vi "CreatActivationCode.vi"() -> ()   [LabVIEW 2018]
panel:
  in  "生成":bool
  in  "激活码":string
  in  "MAC":string
  in  "使用期限":timestamp=timestamp(3629145600 s since 1904-01-01) format="%<%Y%m>T"
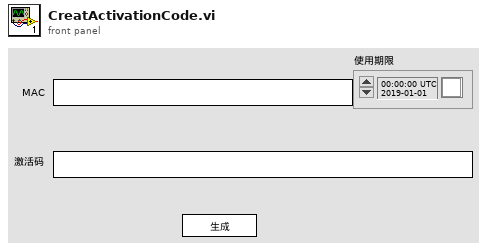
[diagram p1: front panel]
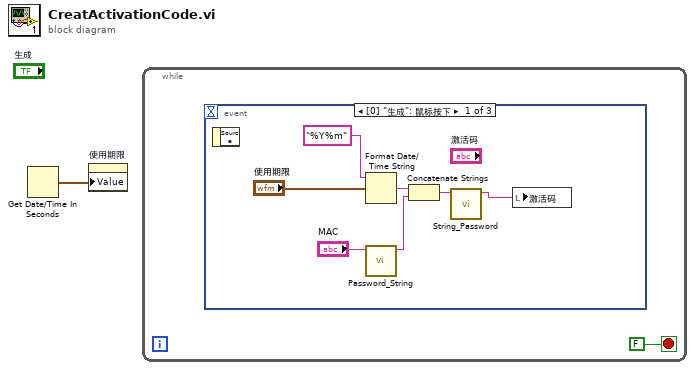
[diagram p0: block diagram]
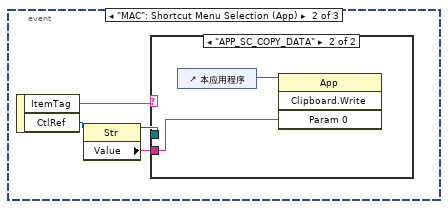
[diagram p2: hidden frame]
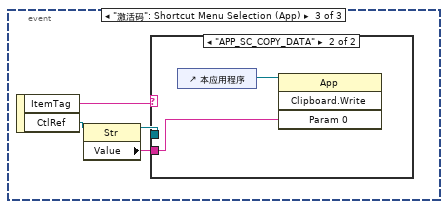
[diagram p4: hidden frame]
diagram:
  n1 = Get Date/Time In Seconds() -> (seconds since 1Jan1904=w1:timestamp)
  n2 = property on="使用期限" class="AbsTime (严格)"("Value"=w1) -> ()  [unwired: 2 in, 2 out]
  n3 = while {
    stop <- FALSE stop-if-true
    n4 = event shown="[0] \"生成\": 鼠标按下" {
      selector: _ -> [_ _ _]
      dyn-events: _ -> [_ _ _]
      timeout: _ -> [_ _ _]
      event "生成": Mouse Down {
        n5 = event-data() -> ()  [unwired: 1 in, 1 out]
        n6 = Format Date/Time String(time format string (%c)="%Y%m" ("时间格式字符串(%c)"), seconds (now)="使用期限") -> (date/time string=w7:string)  [unwired: 1 in]
        n7 = call "Password_String.vi"("Password"="MAC") -> ("String"=w4:string)  [unwired: 10 in]
        n8 = Concatenate Strings(w7, w4) -> (w6:string)
        n9 = call "String_Password.vi"("String"=w6) -> ("Password"=w3:string)  [unwired: 10 in]
        n10 = local write "激活码"(w3) -> ()
      }
      event "MAC": Shortcut Menu Selection (App) {
        n11 = event-data() -> ("ItemTag"=w13:string, "CtlRef"=w12:refnum<vi>)  [unwired: 1 in]
        n12 = property class="Str"(reference=w12) -> (reference out=w10:refnum<vi>, "Value"=w11:string)  [unwired: 1 in, 1 out]
        n13 = case shown="\"APP_SC_COPY_DATA\"" w13 {
          tunnel: w11 -> [_ w14]
          tunnel: w10 -> [_ _]
          frame "假", Default {
          }
          frame "APP_SC_COPY_DATA" {
            n14 = control-ref of="本应用程序"() -> (w15:refnum<vi>)
            n15 = invoke class="App" method="Clipboard.Write"(reference=w15, "Param 0"=w14) -> ()  [unwired: 2 in, 4 out]
          }
        }
      }
      event "激活码": Shortcut Menu Selection (App) {
        n16 = event-data() -> ("ItemTag"=w19:string, "CtlRef"=w18:refnum<vi>)  [unwired: 1 in]
        n17 = property class="Str"(reference=w18) -> (reference out=w16:refnum<vi>, "Value"=w17:string)  [unwired: 1 in, 1 out]
        n18 = case shown="\"APP_SC_COPY_DATA\"" w19 {
          tunnel: w17 -> [_ w20]
          tunnel: w16 -> [_ _]
          frame "假", Default {
          }
          frame "APP_SC_COPY_DATA" {
            n19 = control-ref of="本应用程序"() -> (w21:refnum<vi>)
            n20 = invoke class="App" method="Clipboard.Write"(reference=w21, "Param 0"=w20) -> ()  [unwired: 2 in, 4 out]
          }
        }
      }
    }
  }
